vi "Function.vi"(8 "error in (no error)":errorcluster, 10 "Value":u32, 11 "Two Terminal in":refnum<class "Increment_U32.lvclass">) -> (0 "error out":errorcluster, 2 "Result":u32, 3 "Two Terminal out":refnum<class "Increment_U32.lvclass">)   [LabVIEW 2021, in "Increment_U32.lvclass"]
uses:
  Increment_U32.lvclass
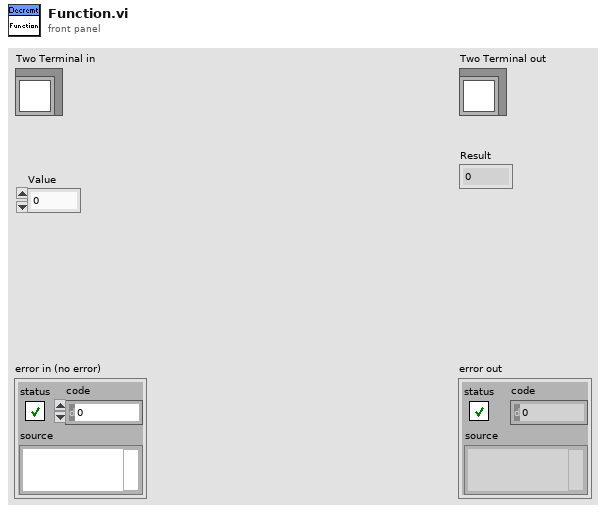
[diagram p1: front panel]
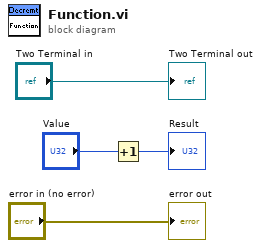
[diagram p0: block diagram]
diagram:
  n1 = Increment(x="Value") -> (x+1=→"Result":u32)
  "error out" <- "error in (no error)"
  "Two Terminal out" <- "Two Terminal in"
